vi "Sub_StairCaseSweep.vi"(0 "Keithley In":refnum<visa-resource-name>, 1 "STSW_Series":T3 {"VSleep/sec" format="%#_13g"; "VStep/V" format="%#_13g"; "VEnd/V" format="%#_13g"; "VStart/V" format="%#_13g"}, 2 "Channel_Series":T2 {"Switch Rate/s" format="%#_13g"}, 3 "Error In":errorcluster, 4 "Halt Ref In":refnum<data-value>) -> (5 "Keithley Out":refnum<visa-resource-name>, 6 "Keithley Feedback":T1, 7 "Error Out":errorcluster)   [LabVIEW 2014]
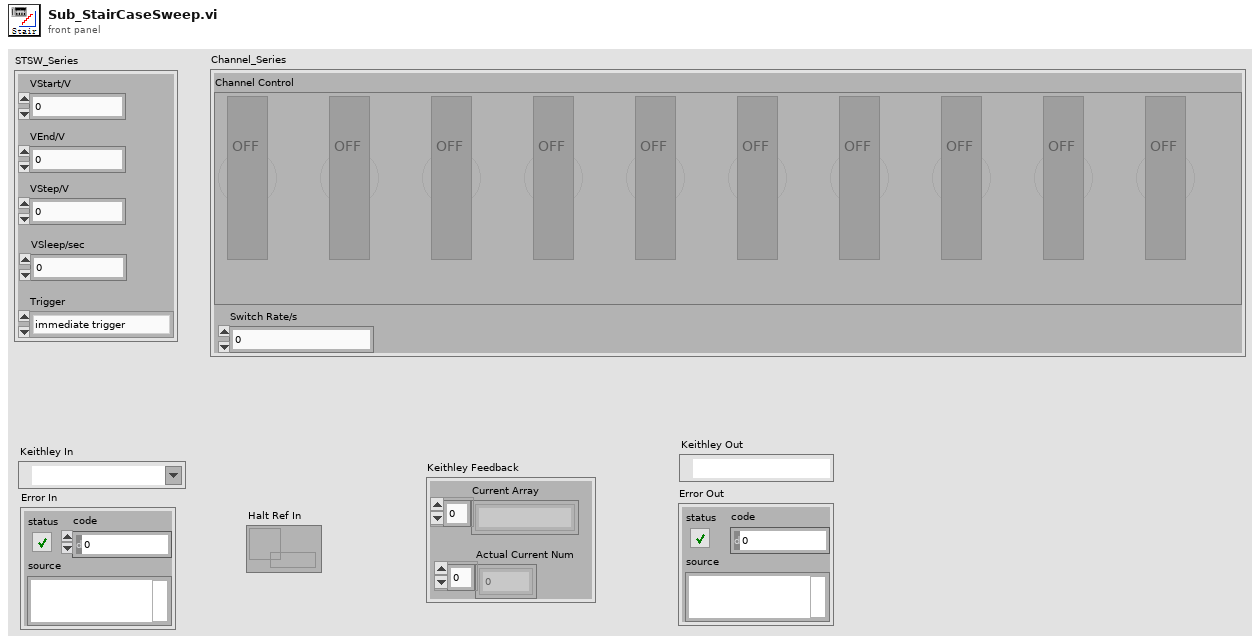
[diagram p1: front panel]
types:
  T1 = cluster{"Current Array":string[], "Actual Current Num":i32[]}
  T2 = cluster{"Channel Control":bool[], "Switch Rate/s":dbl}
  T3 = cluster{"VStart/V":dbl, "VEnd/V":dbl, "VStep/V":dbl, "VSleep/sec":dbl, "Trigger":enum16{"immediate trigger", "delay trigger", "local trigger"}}
  T4 = enum16{"immediate trigger", "delay trigger", "local trigger"}
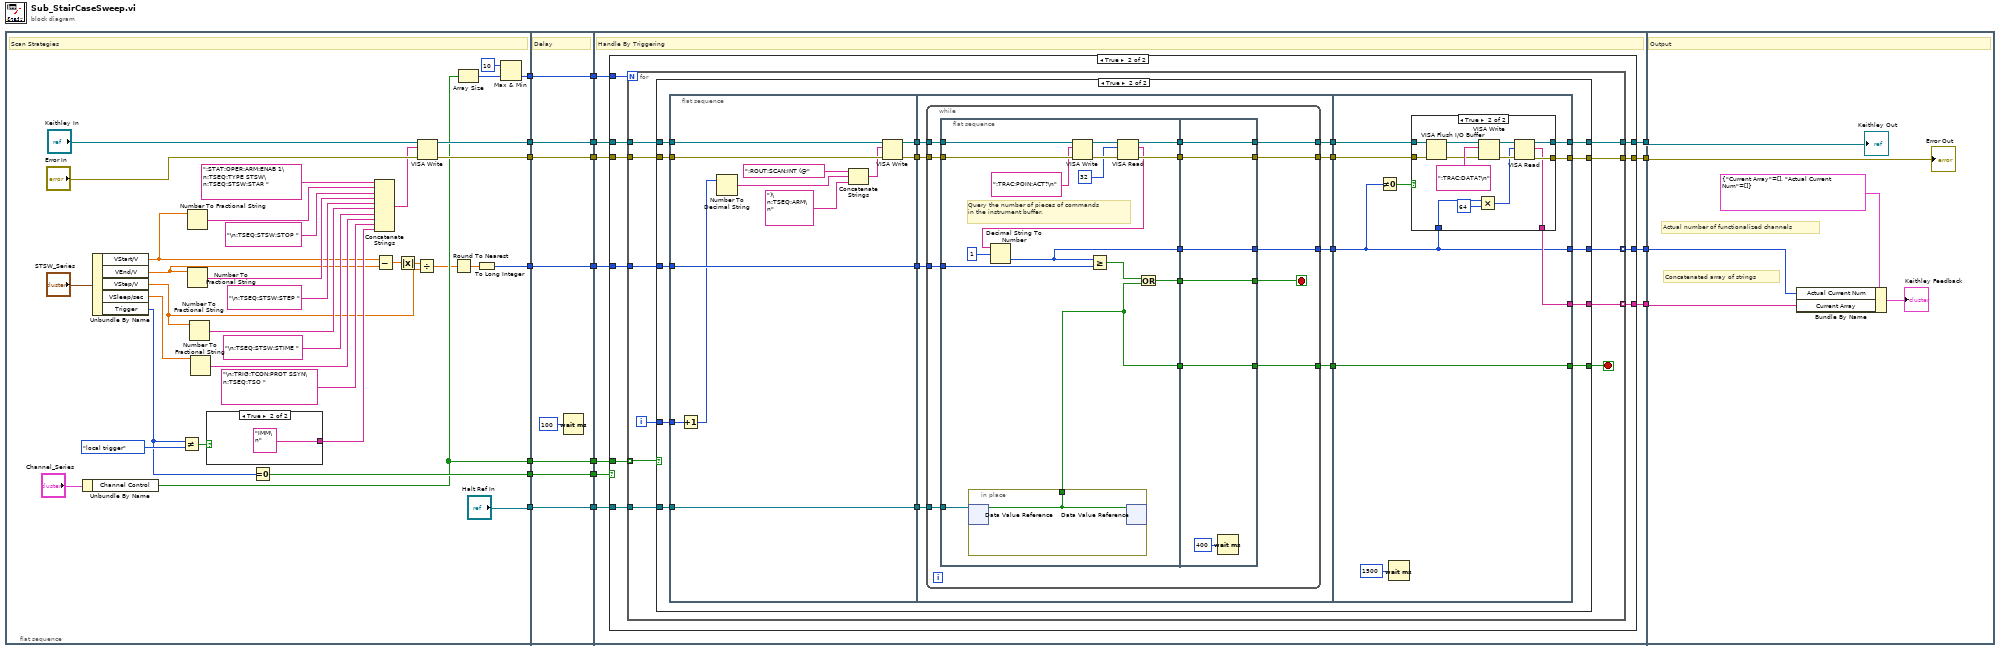
[diagram p0: block diagram]
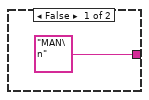
[diagram p2: hidden frame]
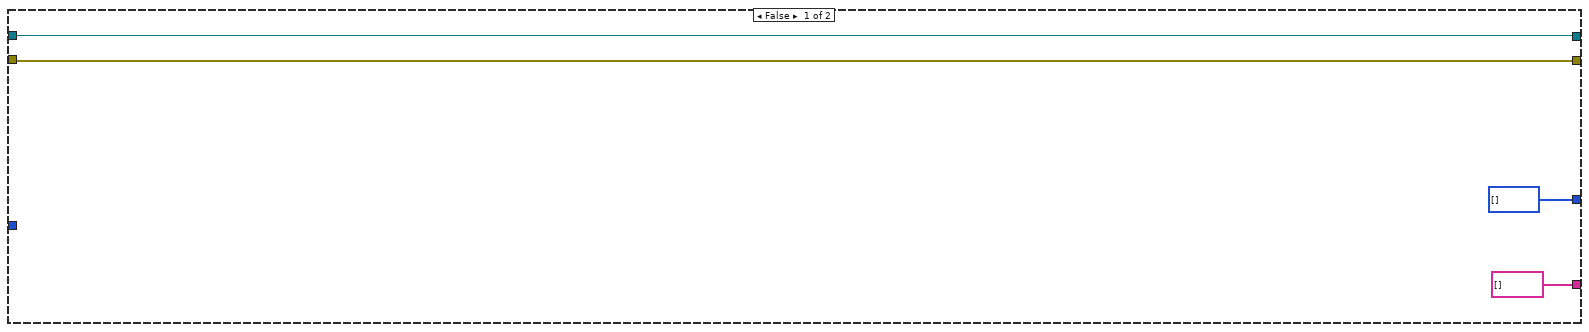
[diagram p3: hidden frame]
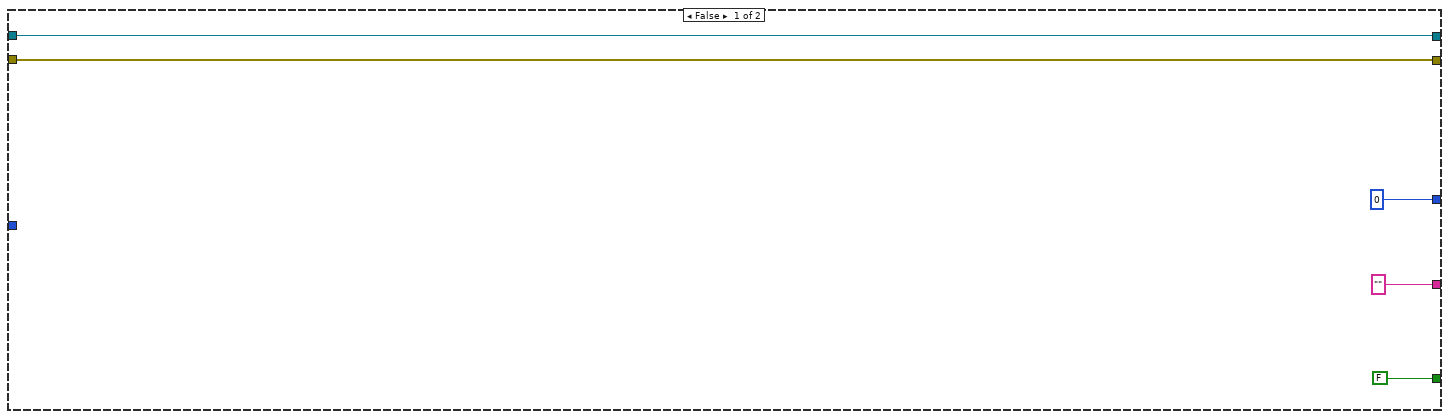
[diagram p4: hidden frame]
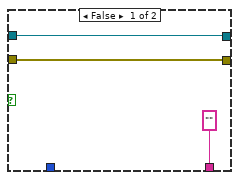
[diagram p5: hidden frame]
diagram:
  n1 = flat-sequence {
    tunnel: [w36] -> w18
    tunnel: [w35] -> w17
    tunnel: [w33] -> w16
    tunnel: [w31] -> w15
    tunnel: [w28] -> w14
    tunnel: [w20] -> w13
    tunnel: ["Halt Ref In"] -> w12
    tunnel: [w62] -> w11
    tunnel: w18 -> [w62]
    tunnel: [w61] -> w10
    tunnel: w17 -> [w61]
    tunnel: [w60] -> w9
    tunnel: w16 -> [w60]
    tunnel: [w59] -> w8
    tunnel: w15 -> [w59]
    tunnel: w14 -> [w58]
    tunnel: [w58] -> w7
    tunnel: [w57] -> w6
    tunnel: w13 -> [w57]
    tunnel: [w56] -> w5
    tunnel: w12 -> [w56]
    tunnel: w11 -> [w72]
    tunnel: w10 -> [w71]
    tunnel: w9 -> [w74]
    tunnel: w8 -> [w73]
    tunnel: w7 -> [w70]
    tunnel: w6 -> [w69]
    tunnel: [w68] -> w4
    tunnel: [w67] -> w3
    tunnel: [w66] -> w2
    tunnel: [w65] -> w1
    tunnel: w5 -> [w64]
    tunnel: w4 -> [w208]
    tunnel: w3 -> [w207]
    tunnel: w2 -> [w206]
    tunnel: w1 -> [w205]
    frame #0 {
      # "Scan Strategies"
      n2 = Unbundle By Name("Channel_Series") -> ("Channel Control"=w28:bool[])
      n3 = Unbundle By Name("STSW_Series") -> ("VStart/V"=w27:dbl, "VEnd/V"=w26:dbl, "VStep/V"=w25:dbl, "VSleep/sec"=w43:dbl, "Trigger"=w34:T4)
      n4 = Not Equal?(x=w34, y=T4."local trigger") -> (x != y?=w40:bool)
      n5 = Number To Fractional String(number=w27) -> (F-format string=w49:string)  [unwired: 3 in]
      n6 = Number To Fractional String(number=w26) -> (F-format string=w47:string)  [unwired: 3 in]
      n7 = Number To Fractional String(number=w25) -> (F-format string=w45:string)  [unwired: 3 in]
      n8 = Number To Fractional String(number=w43) -> (F-format string=w42:string)  [unwired: 3 in]
      n9 = case shown="True" w40 {
        tunnel: ["MAN\n" "IMM\n"] -> w38
        frame False {
        }
        frame True {
        }
      }
      n10 = Equal To 0?(x=w34) -> (x = 0?=w33:bool)
      n11 = Concatenate Strings(":STAT:OPER:ARM:ENAB 1\n:TSEQ:TYPE STSW\n:TSEQ:STSW:STAR " ("string"), w49, "\n:TSEQ:STSW:STOP " ("string"), w47, "\n:TSEQ:STSW:STEP " ("string"), w45, "\n:TSEQ:STSW:STIME " ("string"), w42, "\n:TRIG:TCON:PROT SSYN\n:TSEQ:TSO " ("string"), w38) -> (w37:string)
      n12 = Subtract(x=w27, y=w26) -> (x-y=w23:dbl)
      n13 = Absolute Value(x=w23) -> (abs(x)=w24:dbl)
      n14 = Divide(x=w24, y=w25) -> (x/y=w22:dbl)
      n15 = VISA Write(VISA resource name="Keithley In", write buffer=w37, error in (no error)="Error In") -> (VISA resource name out=w36:refnum<visa-resource-name>, error out=w35:errorcluster)  [unwired: 1 out]
      n16 = Round To Nearest(number=w22) -> (nearest integer value=w21:dbl)
      n17 = Array Size(array=w28) -> (size(s)=w30:i32)
      n18 = To Long Integer(number=w21) -> (32bit integer=w20:i32)
      n19 = Max & Min(x=10, y=w30) -> (min(x,y)=w31:i32)  [unwired: 1 out]
    }
    frame #1 {
      # "Delay"
      n20 = Wait (ms)(milliseconds to wait=u32 100) -> ()  [unwired: 1 out]
    }
    frame #2 {
      # "Handle By Triggering"
      n21 = case shown="True" w74 {
        tunnel: w73 -> [_ w88]
        tunnel: w72 -> [w78 w87]
        tunnel: w71 -> [w77 w86]
        tunnel: w70 -> [_ w85]
        tunnel: w69 -> [_ w84]
        tunnel: [w78 w83] -> w68
        tunnel: [w77 w82] -> w67
        tunnel: [i32[] [] w81] -> w66
        tunnel: [string[] [] w80] -> w65
        tunnel: w64 -> [_ w79]
        frame False {
        }
        frame True {
          n22 = for {
            N: w88 -> [_]
            tunnel: w87 -> [w98]
            tunnel: w86 -> [w97]
            tunnel: w85 -> [w99] mode=indexing
            tunnel: w84 -> [w95]
            tunnel: [w93] -> w83
            tunnel: [w92] -> w82
            tunnel: [w91] -> w81 mode=indexing
            tunnel: [w90] -> w80 mode=indexing
            tunnel: w79 -> [w89]
            i -> [w96]
            stop <- w94 stop-if-true
            n23 = case shown="True" w99 {
              tunnel: w98 -> [w104 w122]
              tunnel: w97 -> [w103 w121]
              tunnel: w96 -> [_ w118]
              tunnel: w95 -> [_ w114]
              tunnel: [FALSE w112] -> w94
              tunnel: [w104 w111] -> w93
              tunnel: [w103 w110] -> w92
              tunnel: [0 w108] -> w91
              tunnel: ["" ("read buffer") w107] -> w90
              tunnel: w89 -> [_ w106]
              frame False {
              }
              frame True {
                n24 = flat-sequence {
                  tunnel: w122 -> [w134]
                  tunnel: w121 -> [w133]
                  tunnel: [w132] -> w120
                  tunnel: [w131] -> w119
                  tunnel: w118 -> [w124]
                  tunnel: [w126] -> w115
                  tunnel: w114 -> [w126]
                  tunnel: w106 -> [w125]
                  tunnel: [w125] -> w105
                  tunnel: w120 -> [w142]
                  tunnel: w119 -> [w141]
                  tunnel: [w140] -> w117
                  tunnel: [w139] -> w116
                  tunnel: w115 -> [w138]
                  tunnel: [w137] -> w113
                  tunnel: [w136] -> w109
                  tunnel: w105 -> [w135]
                  tunnel: w117 -> [w184]
                  tunnel: w116 -> [w183]
                  tunnel: [w187] -> w112
                  tunnel: w113 -> [w187]
                  tunnel: [w186] -> w111
                  tunnel: [w185] -> w110
                  tunnel: w109 -> [w181]
                  tunnel: [w181] -> w108
                  tunnel: [w182] -> w107
                  frame #0 {
                    n25 = Increment(x=w124) -> (x+1=w123:i32)
                    n26 = Number To Decimal String(number=w123) -> (decimal integer string=w129:string)  [unwired: 1 in]
                    n27 = Concatenate Strings(":ROUT:SCAN:INT (@" ("string"), w129, ")\n:TSEQ:ARM\n" ("string")) -> (w127:string)
                    n28 = VISA Write(VISA resource name=w134, write buffer=w127, error in (no error)=w133) -> (VISA resource name out=w132:refnum<visa-resource-name>, error out=w131:errorcluster)  [unwired: 1 out]
                  }
                  frame #1 {
                    n29 = while {
                      tunnel: w142 -> [w156]
                      tunnel: w141 -> [w155]
                      tunnel: [w152] -> w140
                      tunnel: [w151] -> w139
                      tunnel: w138 -> [w150]
                      tunnel: [w146] -> w137
                      tunnel: [w144] -> w136
                      tunnel: w135 -> [w143]
                      stop <- w148 stop-if-true
                      n30 = flat-sequence {
                        tunnel: w156 -> [w172]
                        tunnel: w155 -> [w171]
                        tunnel: [w166] -> w154
                        tunnel: [w165] -> w153
                        tunnel: w150 -> [w162]
                        tunnel: [w159] -> w149
                        tunnel: [w157] -> w147
                        tunnel: [w161] -> w145
                        tunnel: w143 -> [w160]
                        tunnel: w154 -> [w179]
                        tunnel: w153 -> [w178]
                        tunnel: [w179] -> w152
                        tunnel: [w178] -> w151
                        tunnel: [w176] -> w148
                        tunnel: w149 -> [w176]
                        tunnel: [w175] -> w146
                        tunnel: w147 -> [w175]
                        tunnel: [w174] -> w144
                        tunnel: w145 -> [w174]
                        frame #0 {
                          # "Query the number of pieces of commands\nin the instrument buffer."
                          n31 = in-place {
                            in-place-border: [w173] -> w157
                            n32 = in-place-dvr #1(w160) -> (w173:bool)  [unwired: 1 out]
                            n33 = in-place-dvr #1(w173) -> ()  [unwired: 2 out]
                          }
                          n34 = VISA Write(VISA resource name=w172, write buffer=":TRAC:POIN:ACT?\n", error in (no error)=w171) -> (VISA resource name out=w169:refnum<visa-resource-name>, error out=w168:errorcluster)  [unwired: 1 out]
                          n35 = VISA Read(VISA resource name=w169, byte count=u32 32, error in (no error)=w168) -> (VISA resource name out=w166:refnum<visa-resource-name>, read buffer=w164:string, error out=w165:errorcluster)  [unwired: 1 out]
                          n36 = Decimal String To Number(string=w164, offset=1) -> (number=w161:i32)  [unwired: 1 in, 1 out]
                          n37 = Greater Or Equal?(x=w161, y=w162) -> (x >= y?=w158:bool)
                          n38 = Or(x=w158, y=w157) -> (x .or. y?=w159:bool)
                        }
                        frame #1 {
                          n39 = Wait (ms)(milliseconds to wait=u32 400) -> ()  [unwired: 1 out]
                        }
                      }
                    }
                  }
                  frame #2 {
                    n40 = Not Equal To 0?(x=w181) -> (x != 0?=w180:bool)
                    n41 = Wait (ms)(milliseconds to wait=u32 1500) -> ()  [unwired: 1 out]
                    n42 = case shown="True" w180 {
                      tunnel: [w190 w202] -> w186
                      tunnel: [w189 w201] -> w185
                      tunnel: w181 -> [_ w199]
                      tunnel: w184 -> [w190 w196]
                      tunnel: w183 -> [w189 w195]
                      tunnel: ["" ("read buffer") w192] -> w182
                      frame False {
                      }
                      frame True {
                        n43 = VISA Flush I/O Buffer(VISA resource name=w196, error in (no error)=w195) -> (VISA resource name out=w194:refnum<visa-resource-name>, error out=w193:errorcluster)  [unwired: 1 in]
                        n44 = Multiply(x=w199, y=64) -> (x*y=w197:i32)
                        n45 = VISA Write(VISA resource name=w194, write buffer=":TRAC:DATA?\n", error in (no error)=w193) -> (VISA resource name out=w204:refnum<visa-resource-name>, error out=w203:errorcluster)  [unwired: 1 out]
                        n46 = VISA Read(VISA resource name=w204, byte count=w197, error in (no error)=w203) -> (VISA resource name out=w202:refnum<visa-resource-name>, read buffer=w192:string, error out=w201:errorcluster)  [unwired: 1 out]
                      }
                    }
                  }
                }
              }
            }
          }
        }
      }
    }
    frame #3 {
      # "Concatenated array of strings"
      # "Actual number of functionalized channels"
      # "Output"
      n47 = Bundle By Name(cluster=T1 {"Current Array"=[], "Actual Current Num"=[]} ("Keithley Feedback 2"), "Actual Current Num"=w206, "Current Array"=w205) -> (→"Keithley Feedback":T1)
      "Keithley Out" <- w208
      "Error Out" <- w207
    }
  }
